vi "pop.vi"(8 "action list IN":refnum<class "action.lvclass">[](array[class]), 9 "action IN":refnum<class "action.lvclass">, 11 "action stack In":refnum<class "action.lvclass">[](array[class])) -> (1 "action OUT":refnum<class "action.lvclass">, 2 "stack is empty ?":bool, 3 "action stack Out":refnum<class "action.lvclass">[](array[class]))   [LabVIEW 2018, in "action.lvclass"]
uses:
  action.lvclass
  stack action -- control.ctl
  action.lvclass/action.ctl
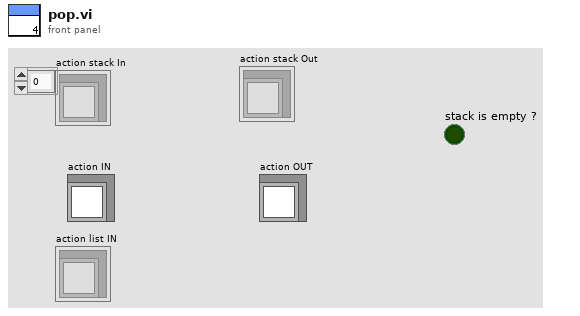
[diagram p1: front panel]
types:
  T1 = typedef "stack action -- control.ctl" = enum16{"push", "pop", "check", "init"}
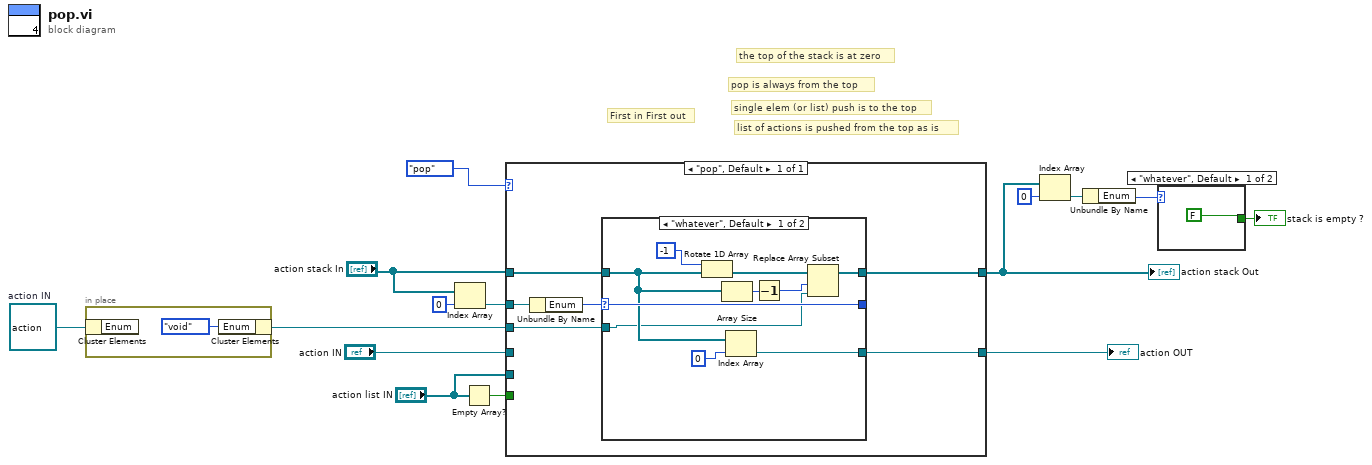
[diagram p0: block diagram]
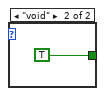
[diagram p2: hidden frame]
diagram:
  w4 = refnum<class "action.lvclass"> refnum  # action IN
  # "list of actions is pushed from the top as is"
  # "single elem (or list) push is to the top"
  # "pop is always from the top"
  # "First in First out"
  # "the top of the stack is at zero"
  n1 = in-place {
    n2 = in-place-cluster #1(w4) -> ()  [unwired: 1 out]
    n3 = in-place-cluster #1("Enum"=enum16{"void", "whatever"}."void") -> (w3:refnum<class "action.lvclass">)
  }
  n4 = Index Array(array="action stack In", index=0) -> (element=w12:refnum<class "action.lvclass">)
  n5 = Empty Array?(array="action list IN") -> (empty?=w14:bool)
  n6 = case shown="\"pop\", Default" stack_action_--_control."pop" ("stack action") {
    tunnel: [w22] -> w6
    tunnel: "action stack In" -> [w21]
    tunnel: w12 -> [w18]
    tunnel: [w20] -> w5
    tunnel: "action IN" -> [_]
    tunnel: w14 -> [_]
    tunnel: "action list IN" -> [_]
    tunnel: w3 -> [w19]
    frame "pop", Default {
      n7 = Unbundle By Name(w18) -> ("Enum"=w17:enum16{"void", "whatever"})
      n8 = case shown="\"whatever\", Default" w17 {
        selector: w17 -> [w30 w34]
        tunnel: [w26 w35] -> w22
        tunnel: w21 -> [w27 w35]
        tunnel: [w31 w33] -> w20
        tunnel: [w30 w34] -> _
        tunnel: w19 -> [w23 w33]
        frame "whatever", Default {
          n9 = Rotate 1D Array(1:w27, 2:-1) -> (0:w25:refnum<class "action.lvclass">[])
          n10 = Array Size(array=w27) -> (size(s)=w28:i32)
          n11 = Index Array(array=w27, index=0) -> (element=w31:refnum<class "action.lvclass">)
          n12 = Decrement(x=w28) -> (x-1=w24:i32)
          n13 = Replace Array Subset(array=w25, new element=w23, index=w24) -> (w26:refnum<class "action.lvclass">[])
        }
        frame "void" {
        }
      }
    }
  }
  "action stack Out" <- w6
  "action OUT" <- w5
  n14 = Index Array(array=w6, index=0) -> (element=w2:refnum<class "action.lvclass">)
  n15 = Unbundle By Name(w2) -> ("Enum"=w1:enum16{"void", "whatever"})
  n16 = case shown="\"whatever\", Default" w1 {
    tunnel: [FALSE TRUE] -> w10
    frame "whatever", Default {
    }
    frame "void" {
    }
  }
  "stack is empty ?" <- w10
